vi "Configure OAuth.vi"(5 "Oauth2 in":refnum<class "Oauth2.lvclass">, 6 "Refresh Token":string, 7 "Exchange Code Server URI":string caption="Exchange Code Server URI (empty: same as Auth Server)", 8 "scopes":string[](array[string]), 9 "Client Secret":string, 10 "Client ID":string, 11 "Authorization Server URI":string) -> (0 "error out":errorcluster, 3 "Oauth2":refnum<class "Oauth2.lvclass">)   [LabVIEW 2020, in "Oauth2.lvclass"]
uses:
  Oauth2.lvclass
  Oauth2.lvclass/Oauth2.ctl
  <vilib>/LabVIEW Open Source Project/OpenURI/uri/URI.lvclass
  OAuthToken/OAuthAccessToken.lvclass
  OAuthToken/OAuth2 Token Element -- enum.ctl
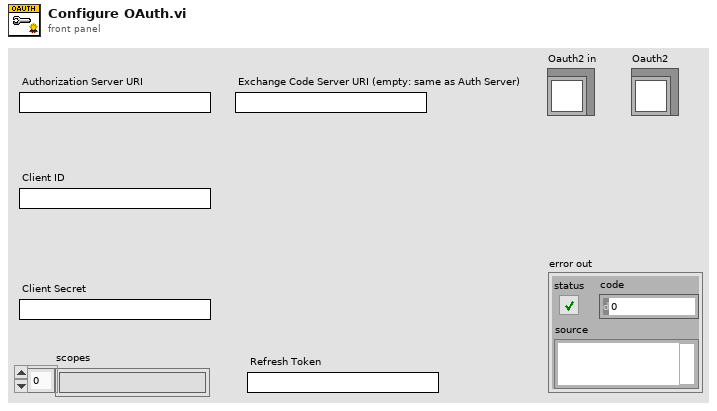
[diagram p1: front panel]
types:
  T1 = typedef "OAuthAccessToken.lvclass/OAuth2 Token Element -- enum.ctl" = enum16{"client_id", "client_secret", "response_type", "scope", "redirect_uri", "error", "error_description", "error_uri", "grant_type", "code", "access_token", "token_type", "expires_in", "username", "password", "refresh_token", "code_challenge", "code_challenge_method", "reverse_proxy_uri", "endpoint element"}
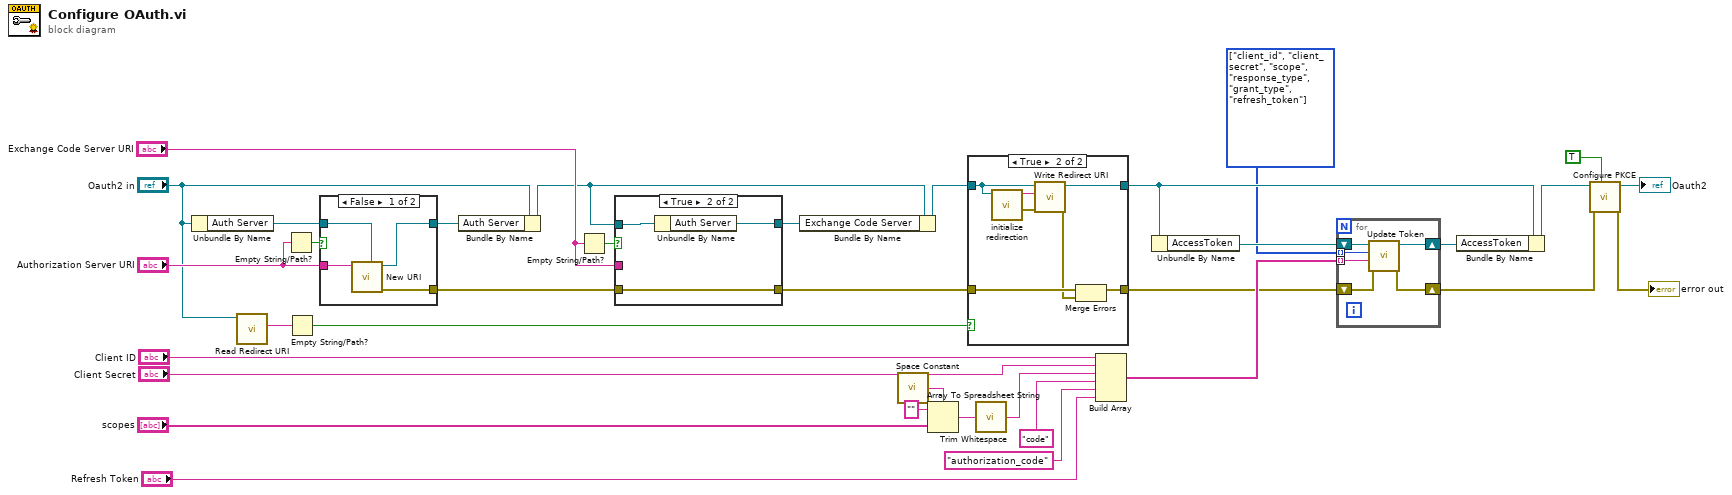
[diagram p0: block diagram]
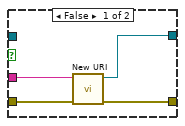
[diagram p2: hidden frame]
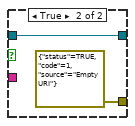
[diagram p3: hidden frame]
diagram:
  w24 = T1[] [enum."client_id", enum."client_secret", enum."scope", enum."response_type", enum."grant_type", enum."refresh_token"] items=["client_id", "client_secret", "response_type", "scope", "redirect_uri", "error", "error_description", "error_uri", "grant_type", "code", "access_token", "token_type", "expires_in", "username", "password", "refresh_token", "code_challenge", "code_challenge_method", "reverse_proxy_uri", "endpoint element"]
  n1 = Unbundle By Name("Oauth2 in") -> ("Auth Server"=w35:refnum<class "URI.lvclass">)
  n2 = call "Read Redirect URI.vi"("Oauth2 in"="Oauth2 in") -> ("Redirect URI"=w16:string)  [unwired: 8 in, 2 out]
  n3 = Empty String/Path?(string/path="Authorization Server URI") -> (empty?=w32:bool)
  n4 = Empty String/Path?(string/path=w16) -> (empty?=w15:bool)
  n5 = case shown="False" w32 {
    tunnel: w35 -> [w39 w41]
    tunnel: [w38 w41] -> w34
    tunnel: "Authorization Server URI" -> [w37 _]
    tunnel: [w36 errorcluster {"status"=TRUE, "code"=1, "source"="Empty URI"} ("error out")] -> w7
    frame False {
      n6 = call <vilib>:"New URI.vi"("URI in"=w39, "URI"=w37) -> ("error out"=w36:errorcluster, "URI"=w38:refnum<class "URI.lvclass">)  [unwired: 8 in]
    }
    frame True {
    }
  }
  n7 = Bundle By Name(cluster="Oauth2 in", "Auth Server"=w34) -> (w1:refnum<class "Oauth2.lvclass">)
  n8 = Empty String/Path?(string/path="Exchange Code Server URI") -> (empty?=w5:bool)
  n9 = case shown="True" w5 {
    tunnel: [w45 w46] -> w3
    tunnel: "Exchange Code Server URI" -> [w44 _]
    tunnel: [w43 w48] -> w6
    tunnel: w7 -> [w42 w48]
    tunnel: w1 -> [_ w47]
    frame False {
      n10 = call <vilib>:"New URI.vi"("error in (no error)"=w42, "URI"=w44) -> ("error out"=w43:errorcluster, "URI"=w45:refnum<class "URI.lvclass">)  [unwired: 8 in]
    }
    frame True {
      n11 = Unbundle By Name(w47) -> ("Auth Server"=w46:refnum<class "URI.lvclass">)
    }
  }
  n12 = Bundle By Name(cluster=w1, "Exchange Code Server"=w3) -> (w2:refnum<class "Oauth2.lvclass">)
  n13 = call <vilib>:"Space Constant.vi"() -> ("String"=w28:string)
  n14 = Array To Spreadsheet String(delimiter (Tab)=w28, array="scopes", 3:"" ("format string")) -> (spreadsheet string=w29:string)
  n15 = case shown="True" w15 {
    tunnel: w2 -> [w50 w54]
    tunnel: [w50 w57] -> w30
    tunnel: [w49 w52] -> w18
    tunnel: w6 -> [w49 w53]
    frame False {
    }
    frame True {
      n16 = call-dynamic "initialize redirection.vi"("Oauth2"=w54) -> ("error out"=w55:errorcluster, "Redirect URI"=w56:string)  [unwired: 9 in]
      n17 = call "Write Redirect URI.vi"("error in (no error)"=w55, "Redirect URI"=w56, "Oauth2 in"=w54) -> ("error out"=w51:errorcluster, "Oauth2 out"=w57:refnum<class "Oauth2.lvclass">)  [unwired: 7 in]
      n18 = Merge Errors(w53, w51) -> (w52:errorcluster)
    }
  }
  n19 = call-poly <vilib>:"Trim Whitespace.vi"("string"=w29) -> ("trimmed string"=w20:string)  [unwired: 1 in]
  n20 = Build Array("Client ID", "Client Secret", w20, "code" ("argument"), "authorization_code" ("argument"), "Refresh Token") -> (w21:string[])
  n21 = Unbundle By Name(w30) -> ("AccessToken"=w31:refnum<class "OAuthAccessToken.lvclass">)
  n22 = for {
    tunnel: w21 -> [w62] mode=indexing
    shift-right: [w61] -> w25
    shift-left: w31 -> [w63]
    tunnel: w24 -> [w60] mode=indexing
    shift-right: [w58] -> w9
    shift-left: w18 -> [w59]
    n23 = call "Update Token.vi"("error in (no error)"=w59, "Value"=w62, "Token element"=w60, "OAuthAccessToken in"=w63) -> ("error out"=w58:errorcluster, "OAuthAccessToken out"=w61:refnum<class "OAuthAccessToken.lvclass">)  [unwired: 6 in]
  }
  n24 = Bundle By Name(cluster=w30, "AccessToken"=w25) -> (w12:refnum<class "Oauth2.lvclass">)
  n25 = call "Configure PKCE.vi"("Use PKCE? (T)"=TRUE, "error in"=w9, "Oauth2 in"=w12) -> ("error out"=→"error out":errorcluster, "Oauth2"=→"Oauth2":refnum<class "Oauth2.lvclass">)  [unwired: 7 in]
